vi "E3-4.vi"() -> ()   [LabVIEW 2011]
panel:
  out "불리언":bool
  out "섭씨 온도":dbl
  in  "화씨 온도":dbl
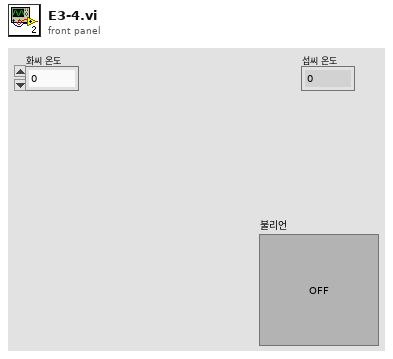
[diagram p1: front panel]
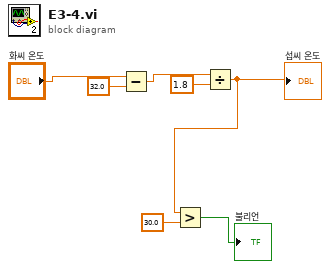
[diagram p0: block diagram]
diagram:
  n1 = Subtract(x="화씨 온도", y=32.0) -> (x-y=w6:dbl)
  n2 = Divide(x=w6, y=1.8) -> (x/y=w3:dbl)
  "섭씨 온도" <- w3
  n3 = Greater?(x=w3, y=30.0) -> (0:→"불리언":bool)
